vi "GlobalIBackImgHndl.vi"() -> ()   [LabVIEW 2010]
panel:
  in  "Back Active data":bool
  in  "Back Image Handle":u32
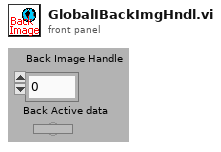
[diagram p1: front panel]
diagram:
